vi "Client.vi"() -> ()   [LabVIEW 2014]
doc: "Demonstrates how to open a connection to an TCP server, read the data being sent, and display the data on a chart. This VI is designed to stop if the TCP connection is terminated."
uses:
  <vilib>/sound2/lvsound2.llb/Sound Output Write (DBL).vi
panel:
  out "data out 2":string
  in  "Stop":bool
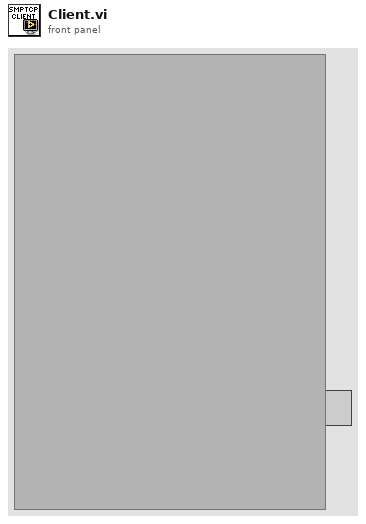
[diagram p1: front panel]
types:
  T1 = typedef "Sound Output Task ID.ctl" = u32
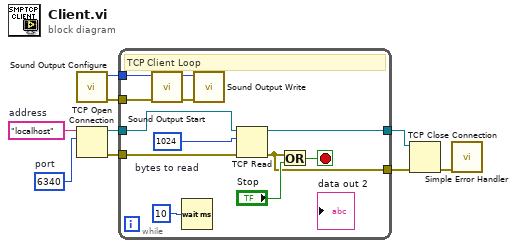
[diagram p0: block diagram]
diagram:
  w5 = u16 6340  # port
  w6 = "localhost"  # address
  n1 = call <vilib>:"Sound Output Configure.vi"() -> ("error out"=w1:errorcluster, "task ID"=w2:T1)  [unwired: 10 in]
  n2 = TCP Open Connection(address=w6, remote port or service name=w5) -> (connection ID=w9:refnum<k5>, error out=w8:errorcluster)  [unwired: 3 in]
  n3 = while {
    tunnel: w8 -> [w16]
    tunnel: w9 -> [w15]
    tunnel: [w17] -> w3
    tunnel: [w18] -> w4
    tunnel: w2 -> [w12]
    tunnel: w1 -> [w11]
    stop <- w20 stop-if-true
    w14 = 1024  # bytes to read
    # "TCP Client Loop"
    n4 = call <vilib>:"Sound Output Start.vi"("error in (no error)"=w11, "task ID"=w12) -> ("error out"=w10:errorcluster, "task ID out"=w13:T1)  [unwired: 8 in]
    n5 = Wait (ms)(milliseconds to wait=u32 10) -> ()  [unwired: 1 out]
    n6 = call-poly <vilib>:"Sound Output Write.vi"("error in (no error)"=w10, "task ID"=w13) -> ()  [unwired: 8 in, 2 out]
    n7 = TCP Read(connection ID=w15, bytes to read=w14, error in (no error)=w16) -> (connection ID out=w17:refnum<k5>, error out=w18:errorcluster)  [unwired: 2 in, 1 out]
    n8 = Or(x=w18, y="Stop") -> (x .or. y?=w20:bool)
  }
  n9 = TCP Close Connection(connection ID=w3, error in (no error)=w4) -> (error out=w7:errorcluster)  [unwired: 1 in, 1 out]
  n10 = call <vilib>:"Simple Error Handler.vi"("error in (no error)"=w7) -> ()  [unwired: 4 in, 5 out]
